vi "Handle Video Image.vi"(4 "queue in":refnum<queue>, 5 "Event Data":cluster{"sender":refnum<k24>, "e":refnum<k24>}, 6 "Control Ref":refnum<k24>, 7 "Event Common Data":T1) -> ()   [LabVIEW 2010]
uses:
  Microsoft.Research.Kinect
  <vilib>/vision/Image Controls.llb/IMAQ Image.ctl
  <vilib>/vision/NI_Vision_Development_Module.lvlib
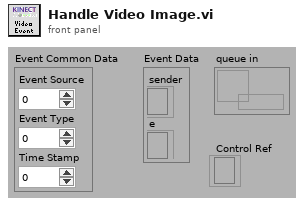
[diagram p1: front panel]
types:
  T1 = cluster{"Event Source":i32, "Event Type":u32, "Time Stamp":u32}
  T2 = typedef "Image Type" = u32
  T3 = typedef "IMAQ Image.ctl" = refnum<image>
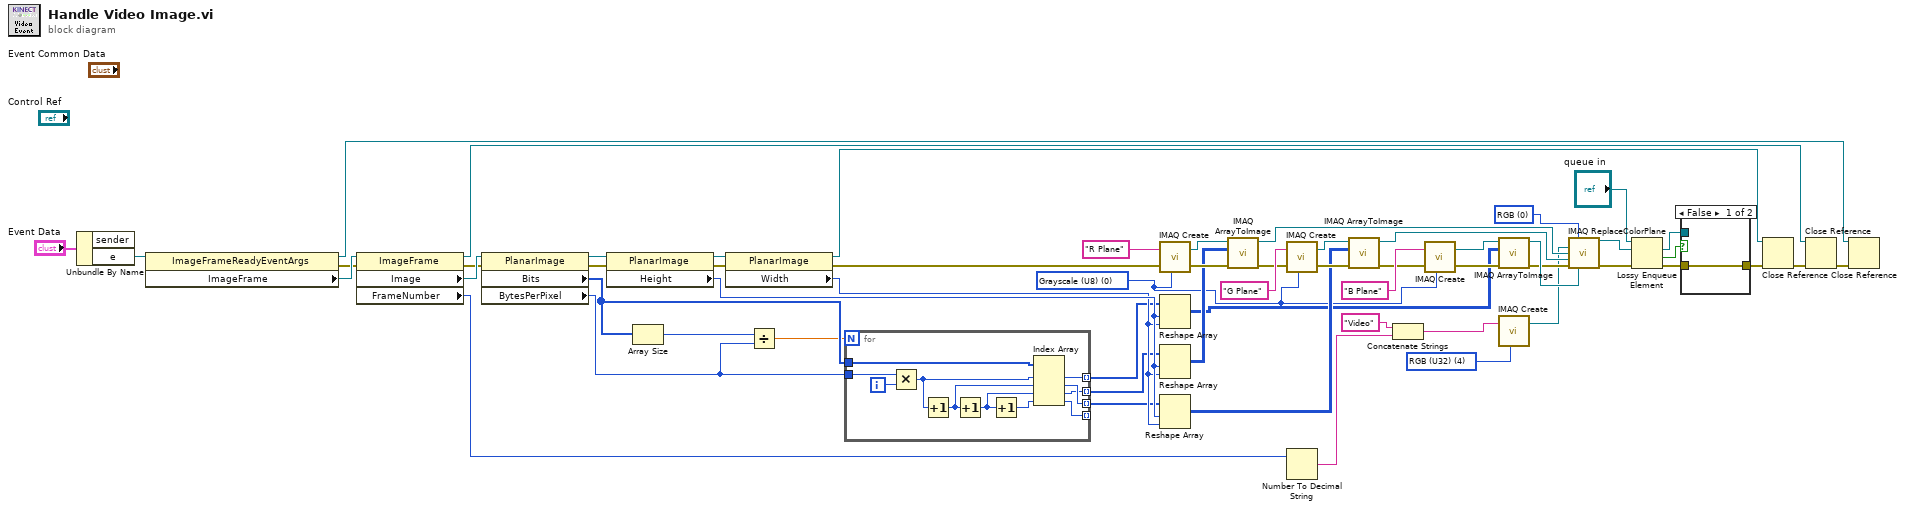
[diagram p0: block diagram]
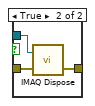
[diagram p2: hidden frame]
diagram:
  w7 = T2 4 items=["Grayscale (U8)", "Grayscale (I16)", "Grayscale (SGL)", "Complex (CSG)", "RGB (U32)", "HSL (U32)", "RGB (U64)", "Grayscale (U16)"] ("Image Type")
  w8 = T2 0 items=["Grayscale (U8)", "Grayscale (I16)", "Grayscale (SGL)", "Complex (CSG)", "RGB (U32)", "HSL (U32)", "RGB (U64)", "Grayscale (U16)"] ("Image Type")
  w31 = u16 0 items=["RGB", "HSL", "HSV", "HSI"] ("Color Mode")
  n1 = Unbundle By Name("Event Data") -> ("e"=w58:refnum<k24>)  [unwired: 1 out]
  n2 = property class="ImageFrameReadyEventArgs"(reference=w58) -> (reference out=w47:refnum<k24>, error out=w44:errorcluster, "ImageFrame"=w57:refnum<k24>)  [unwired: 1 in]
  n3 = property class="ImageFrame"(reference=w57, error in=w44) -> (reference out=w48:refnum<k24>, error out=w45:errorcluster, "Image"=w51:refnum<k24>, "FrameNumber"=w12:i32)
  n4 = property class="PlanarImage"(reference=w51, error in=w45) -> (reference out=w54:refnum<k24>, error out=w56:errorcluster, "Bits"=w27:u8[], "BytesPerPixel"=w24:i32)
  n5 = property class="PlanarImage"(reference=w54, error in=w56) -> (reference out=w52:refnum<k24>, error out=w55:errorcluster, "Height"=w23:i32)
  n6 = Array Size(array=w27) -> (size(s)=w26:i32)
  n7 = property class="PlanarImage"(reference=w52, error in=w55) -> (reference out=w53:refnum<k24>, error out=w5:errorcluster, "Width"=w22:i32)
  n8 = Divide(x=w26, y=w24) -> (x/y=w25:dbl)
  n9 = for {
    N: w25 -> [_]
    tunnel: w27 -> [w64]
    tunnel: [w63] -> w16 mode=indexing
    tunnel: [w62] -> w21 mode=indexing
    tunnel: [w61] -> w17 mode=indexing
    tunnel: [w60] -> _ mode=indexing
    tunnel: w24 -> [w59]
    i -> [w69]
    n10 = Multiply(x=w59, y=w69) -> (x*y=w68:i32)
    n11 = Increment(x=w68) -> (x+1=w67:i32)
    n12 = Increment(x=w67) -> (x+1=w66:i32)
    n13 = Increment(x=w66) -> (x+1=w65:i32)
    n14 = Index Array(array=w64, index #1=w68, index #2=w67, index #3=w66, index #4=w65) -> (element #1=w63:u8, element #2=w62:u8, element #3=w61:u8, element #4=w60:u8)
  }
  n15 = call "IMAQ Create"("Image Name"="R Plane", "Image Type"=w8, "error in (no error)"=w5) -> ("New Image"=w41:T3, "error out"=w40:errorcluster)  [unwired: 2 in]
  n16 = Reshape Array(w16, w23, w22) -> (w18:u8[][])
  n17 = Reshape Array(w17, w23, w22) -> (w20:u8[][])
  n18 = Reshape Array(w21, w23, w22) -> (w19:u8[][])
  n19 = call "IMAQ ArrayToImage"("error in (no error)"=w40, "Image Pixels (U8)"=w20, "Image"=w41) -> ("error out"=w30:errorcluster, "Image Out"=w34:T3)  [unwired: 7 in]
  n20 = call "IMAQ Create"("Image Name"="G Plane", "Image Type"=w8, "error in (no error)"=w30) -> ("New Image"=w42:T3, "error out"=w43:errorcluster)  [unwired: 2 in]
  n21 = Number To Decimal String(number=w12) -> (decimal integer string=w11:string)  [unwired: 1 in]
  n22 = call "IMAQ ArrayToImage"("error in (no error)"=w43, "Image Pixels (U8)"=w19, "Image"=w42) -> ("error out"=w29:errorcluster, "Image Out"=w33:T3)  [unwired: 7 in]
  n23 = Concatenate Strings("Video" ("string"), w11) -> (w10:string)
  n24 = call "IMAQ Create"("Image Name"="B Plane", "Image Type"=w8, "error in (no error)"=w29) -> ("New Image"=w39:T3, "error out"=w38:errorcluster)  [unwired: 2 in]
  n25 = call "IMAQ ArrayToImage"("error in (no error)"=w38, "Image Pixels (U8)"=w18, "Image"=w39) -> ("error out"=w28:errorcluster, "Image Out"=w32:T3)  [unwired: 7 in]
  n26 = call "IMAQ Create"("Image Name"=w10, "Image Type"=w7) -> ("New Image"=w13:T3)  [unwired: 3 in, 1 out]
  n27 = call "IMAQ ReplaceColorPlane"("Color Mode"=w31, "Image Dst"=w13, "Red or Hue Plane"=w34, "Green or Sat Plane"=w33, "error in (no error)"=w28, "Blue or Luma or Val or Inten Plane"=w32) -> ("Image Dst Out"=w15:T3, "error out"=w14:errorcluster)  [unwired: 8 in]
  n28 = Lossy Enqueue Element(queue="queue in", element=w15, error in (no error)=w14) -> (overflow element=w4:T3, overflow?=w1:bool, error out=w3:errorcluster)  [unwired: 1 out]
  n29 = case shown="False" w1 {
    tunnel: w4 -> [_ w73]
    tunnel: w3 -> [w70 w72]
    tunnel: [w70 w71] -> w2
    frame False {
    }
    frame True {
      n30 = call "IMAQ Dispose"("Image"=w73, "error in (no error)"=w72) -> ("error out"=w71:errorcluster)  [unwired: 4 in]
    }
  }
  n31 = Close Reference(reference=w53, error in (no error)=w2) -> (error out=w50:errorcluster)
  n32 = Close Reference(reference=w48, error in (no error)=w50) -> (error out=w49:errorcluster)
  n33 = Close Reference(reference=w47, error in (no error)=w49) -> ()  [unwired: 1 out]
